vi "OpenFile.vi"(8 "error in (no error)":errorcluster, 10 "Path":path) -> (0 "error out":errorcluster, 3 "FileHandler out":refnum<class "FileHandler.lvclass">)   [LabVIEW 2021, in "FileHandler.lvclass"]
uses:
  FileHandler.lvclass
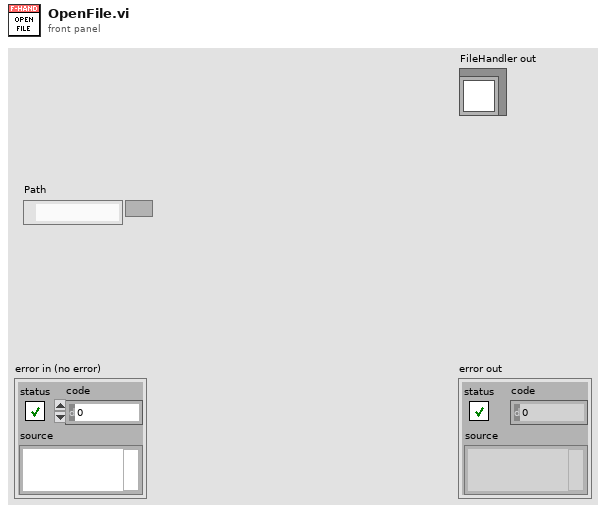
[diagram p1: front panel]
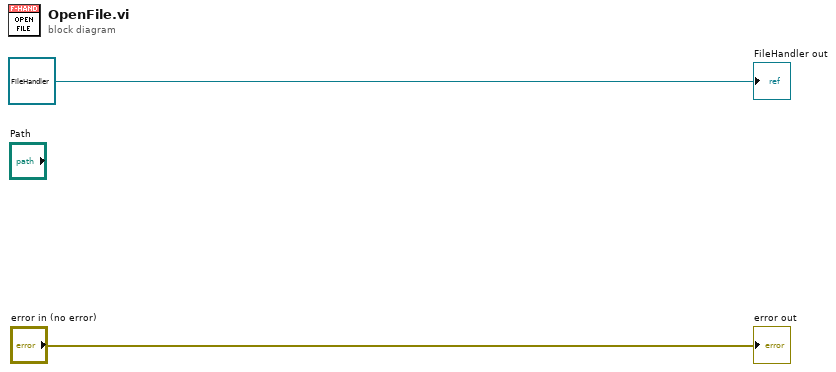
[diagram p0: block diagram]
diagram:
  "error out" <- "error in (no error)"
  "FileHandler out" <- refnum<class "FileHandler.lvclass"> refnum ("FileHandler in")
